vi "Get Mediator.vi"(8 "error in (no error)":errorcluster caption="错误输入（无错误）", 11 "Colleague输入":refnum<class "Colleague.lvclass">) -> (0 "error out":errorcluster caption="错误输出", 2 "Mediator":string, 3 "Colleague输出":refnum<class "Colleague.lvclass">)   [LabVIEW 2011, in "Colleague.lvclass"]
uses:
  Colleague.lvclass
  Colleague.lvclass/Colleague.ctl
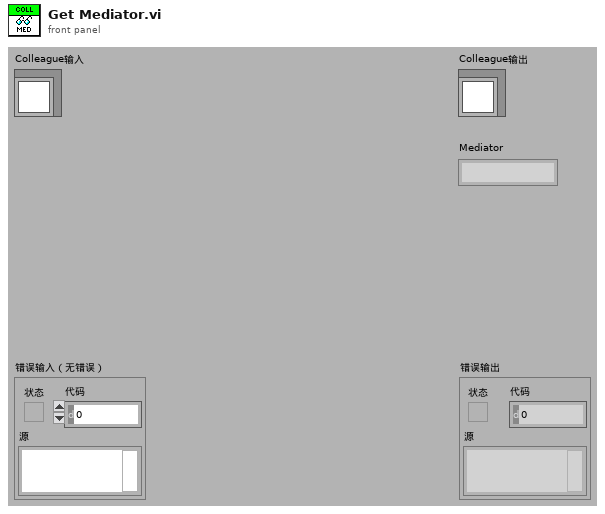
[diagram p1: front panel]
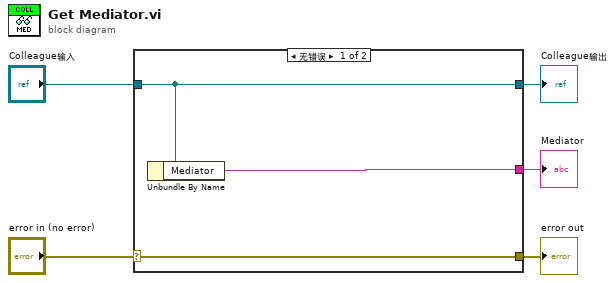
[diagram p0: block diagram]
diagram:
  n1 = case shown="无错误" "error in (no error)" {
    selector: "error in (no error)" -> [w8 w9]
    tunnel: [w8 w9] -> w4
    tunnel: [w7 w10] -> w2
    tunnel: "Colleague输入" -> [w7 w10]
    tunnel: [w6 _] -> w1
    frame No Error {
      n2 = Unbundle By Name(w7) -> ("Mediator"=w6:string)
    }
    frame Error {
    }
  }
  "error out" <- w4
  "Colleague输出" <- w2
  "Mediator" <- w1
